vi "Parse Autonomous (Mark Siekmeier's conflicted copy 2013-04-30).vi"() -> ()   [LabVIEW 2012]
uses:
  Robot Global Data.vi
  Parse CSV From cRIO.vi
panel:
  out "Loop Time 2":u32(graph)
  out "Parsed Array":dbl[][](array[numeric])
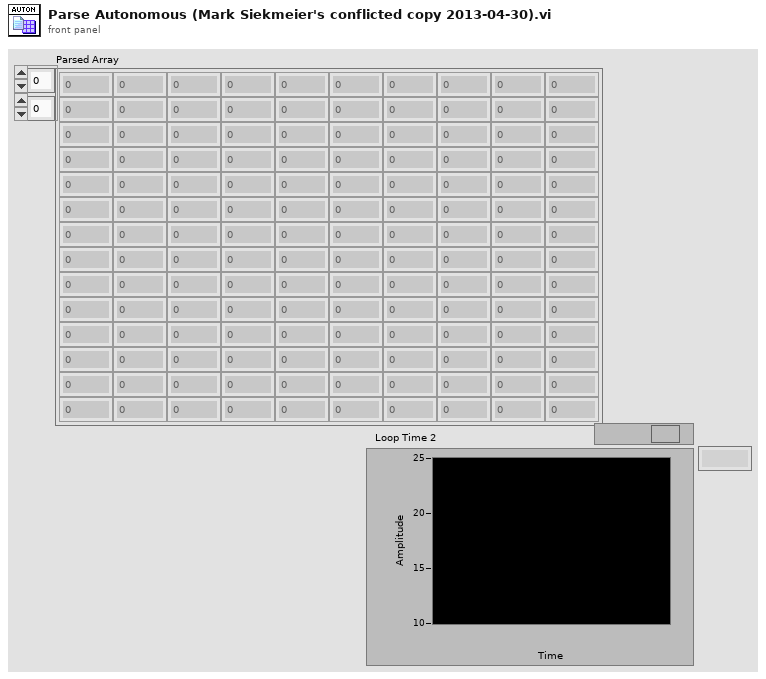
[diagram p1: front panel]
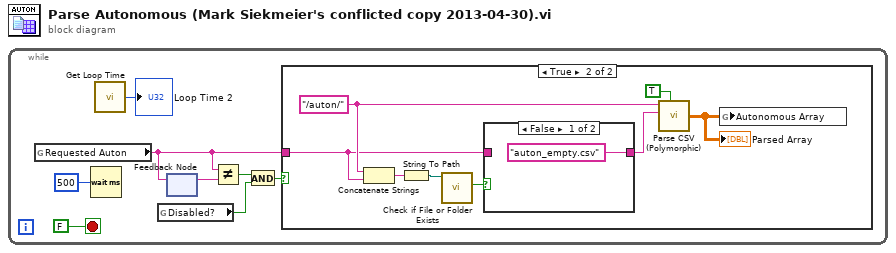
[diagram p0: block diagram]
diagram:
  n1 = while {
    stop <- FALSE stop-if-true
    n2 = global read "Robot Global Data.vi" "Requested Auton"() -> (w7:string)
    n3 = Wait (ms)(milliseconds to wait=u32 500) -> ()  [unwired: 1 out]
    n4 = call "Get Loop Time.vi"() -> ("Loop Time"=→"Loop Time 2":u32)  [unwired: 1 in]
    n5 = global read "Robot Global Data.vi" "Disabled?"() -> (w2:bool)
    n6 = feedback-in #1(w7) -> ()
    n7 = feedback #1() -> (w6:string)  [unwired: 1 in]
    n8 = Not Equal?(x=w7, y=w6) -> (x != y?=w3:bool)
    n9 = And(x=w3, y=w2) -> (x .and. y?=w4:bool)
    n10 = case shown="True" w4 {
      tunnel: w7 -> [_ w9]
      frame False {
      }
      frame True {
        w11 = "/auton/" ("string")
        n11 = Concatenate Strings(w11, w9) -> (w12:string)
        n12 = String To Path(string=w12) -> (path=w14:path)
        n13 = call <vilib>:"Check if File or Folder Exists.vi"("path"=w14) -> ("file or folder exists?"=w13:bool)  [unwired: 8 in, 2 out]
        n14 = case shown="False" w13 {
          tunnel: ["auton_empty.csv" ("string") w18] -> w16
          tunnel: w9 -> [_ w18]
          frame False {
          }
          frame True {
          }
        }
        n15 = call-poly "Parse CSV (Polymorphic).vi"("/path/"=w11, "File Name"=w16, "Header Row?"=TRUE) -> ("Output Array"=w10:dbl[][])  [unwired: 2 in]
        "Parsed Array" <- w10
        n16 = global write "Robot Global Data.vi" "Autonomous Array"(w10) -> ()
      }
    }
  }
